vi "与副屏通信master.vi"() -> ()   [LabVIEW 2016, in "斯坦道多参数.lvlib"]
uses:
  <vilib>/NI/Modbus Library/API/Wrapper/Create TCP Master.vi
  <vilib>/NI/Modbus Library/API/master/Modbus Master.lvclass
  <vilib>/NI/Modbus Library/API/Wrapper/API Main.lvlib
  <vilib>/ptbypt/NI_PtbyPt.lvlib
panel:
  out "副屏启动命令":u16
  in  "停止 2":bool
  out "read values 2":u16[](array[numeric])
  in  "registers to write 2":u16[](array[numeric])
  out "error out 2":errorcluster caption="error out"
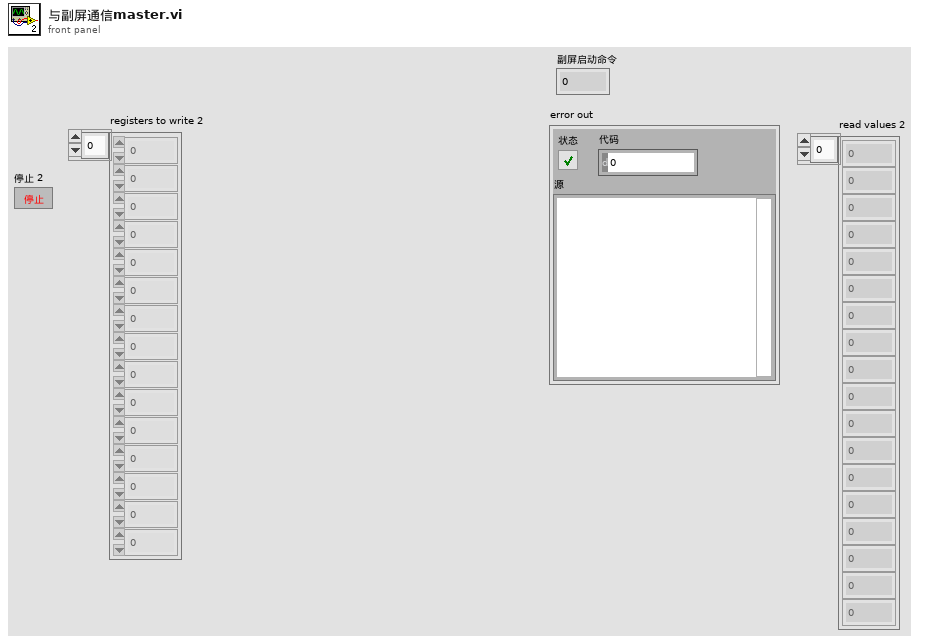
[diagram p1: front panel]
types:
  T1 = enum32{"Bad", "Idle", "Run top level", "Running"}
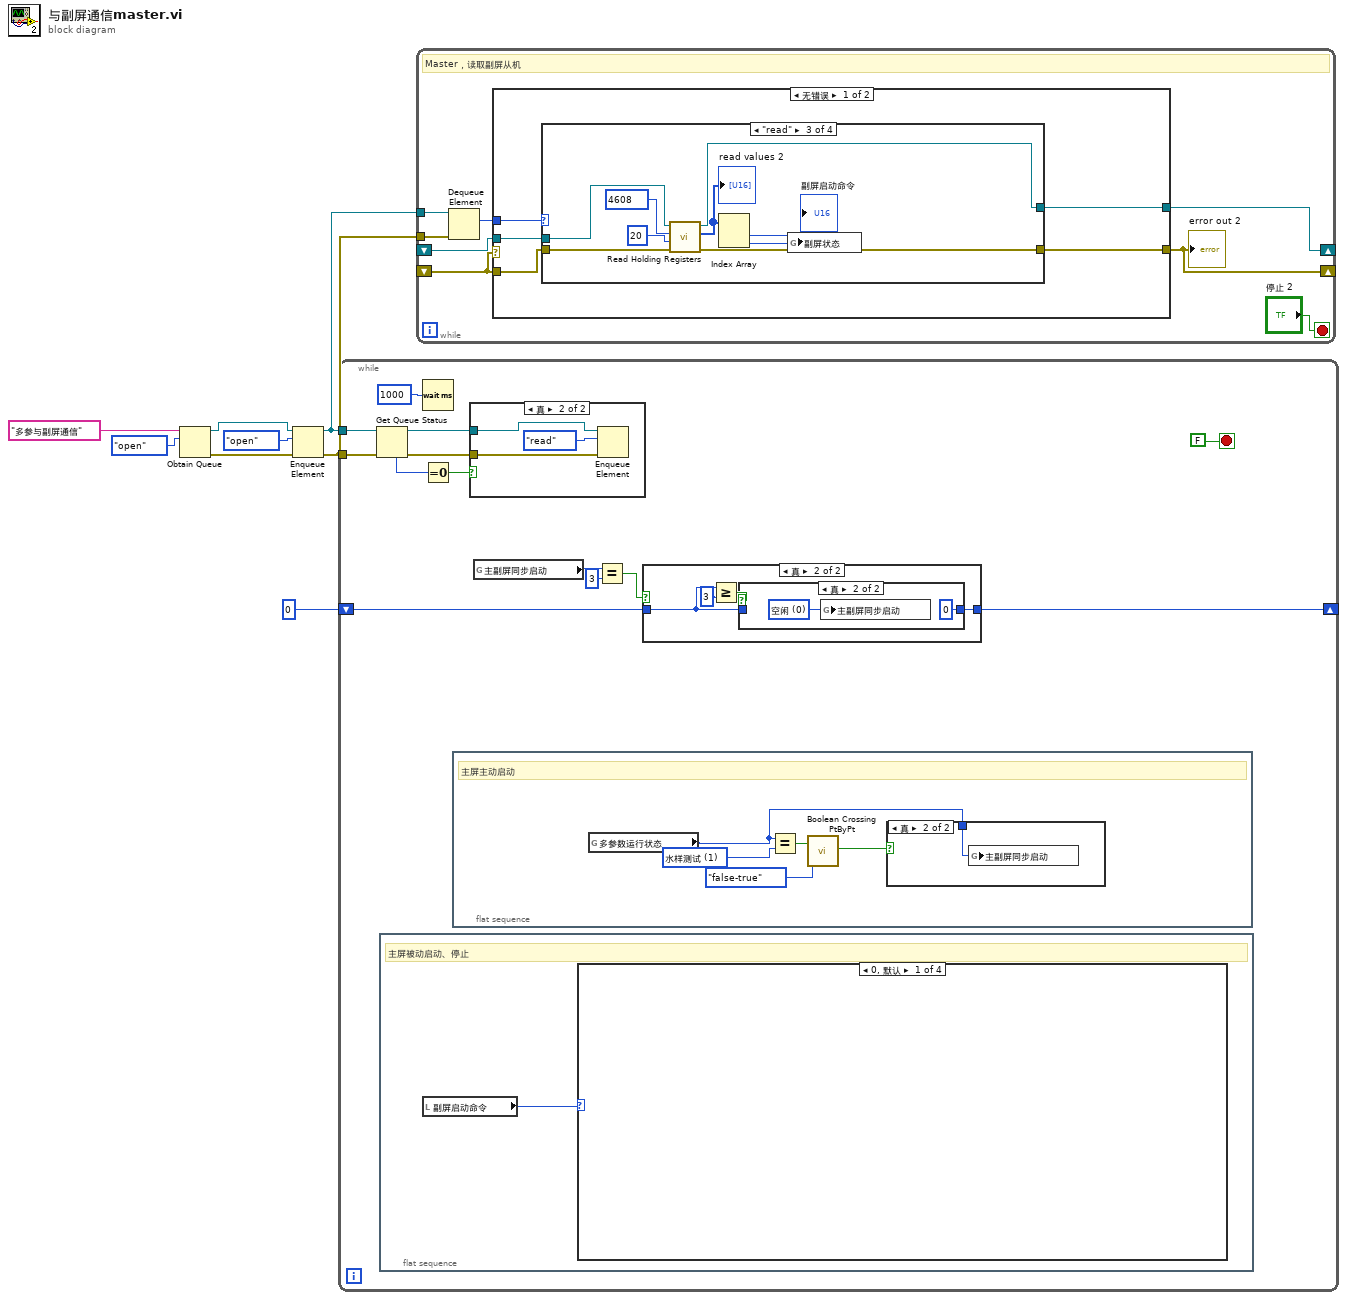
[diagram p0: block diagram]
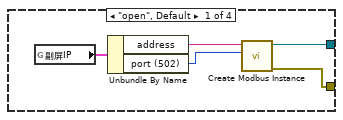
[diagram p2: hidden frame]
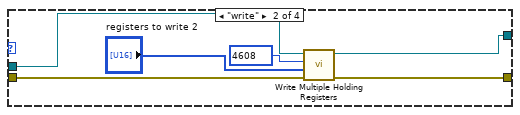
[diagram p3: hidden frame]
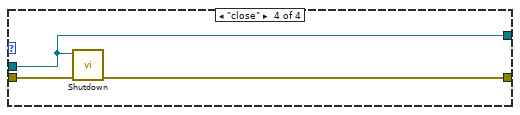
[diagram p4: hidden frame]
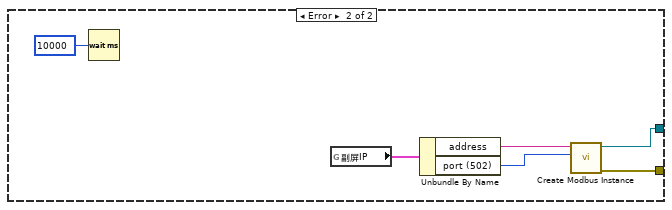
[diagram p5: hidden frame]
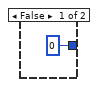
[diagram p6: hidden frame]
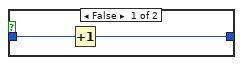
[diagram p7: hidden frame]
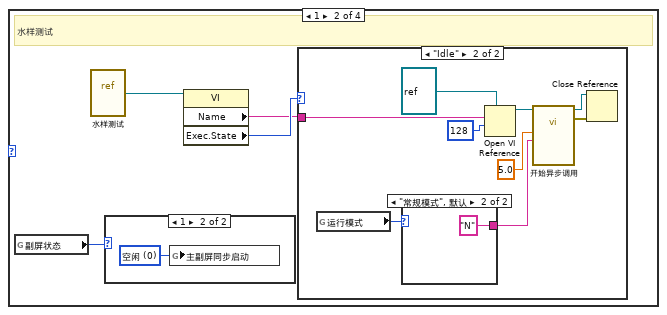
[diagram p8: hidden frame]
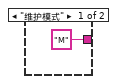
[diagram p11: hidden frame]
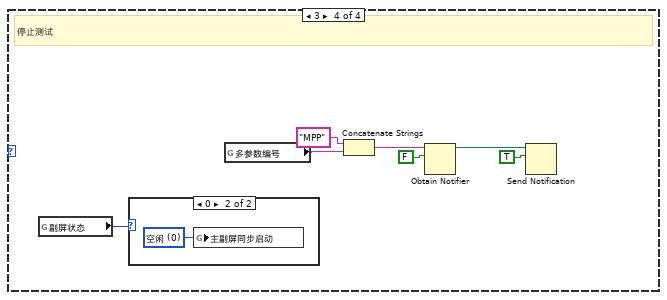
[diagram p13: hidden frame]
diagram:
  n1 = Obtain Queue(name (unnamed)="多参与副屏通信" ("名称（未命名）"), element data type=enum16{"open", "write", "read", "close"}."open") -> (queue out=w5:refnum<queue>, error out=w6:errorcluster)  [unwired: 3 in, 1 out]
  n2 = Enqueue Element(queue=w5, element=enum16{"open", "write", "read", "close"}."open", error in (no error)=w6) -> (queue out=w3:refnum<queue>, error out=w2:errorcluster)  [unwired: 1 in, 1 out]
  n3 = while {
    tunnel: w3 -> [w15]
    tunnel: w2 -> [w14]
    shift-right: [w9] -> _
    shift-left: u32 0 ("等待时间（毫秒）") -> [w10]
    stop <- FALSE stop-if-true
    n4 = Get Queue Status(queue=w15, error in (no error)=w14) -> (queue out=w17:refnum<queue>, error out=w18:errorcluster, # elements in queue=w16:i32)  [unwired: 1 in, 5 out]
    n5 = flat-sequence {
      frame #0 {
        # "主屏被动启动、停止"
        n6 = local read "副屏启动命令"() -> (w31:u16)
        n7 = case shown="0, 默认" w31 {
          frame 0, Default {
          }
          frame 1 {
            # "水样测试"
            n8 = global read "多参数全局变量.vi" "副屏状态"() -> (w32:u16)
            n9 = vi-ref "水样测试.vi"() -> (w35:refnum<vi>)
            n10 = case shown="1" w32 {
              frame 0, Default {
              }
              frame 1 {
                w36 = u16 0 items=["空闲", "水样测试", "标样核查", "停止"] ("主副屏同步启动")
                n11 = global write "多参数全局变量.vi" "主副屏同步启动"(w36) -> ()
              }
            }
            n12 = property class="VI"(reference=w35) -> ("Name"=w33:string, "Exec.State"=w34:T1)  [unwired: 1 in, 2 out]
            n13 = case shown="\"Idle\"" w34 {
              tunnel: w33 -> [_ w42]
              frame "Bad", Default {
              }
              frame "Idle" {
                n14 = global read "多参数全局变量.vi" "运行模式"() -> (w38:enum16{"维护模式", "常规模式", "应急模式", "质控模式"})
                n15 = case shown="\"常规模式\", 默认" w38 {
                  tunnel: ["M" ("数据标记表") "N" ("数据标记表")] -> w37
                  frame "维护模式" {
                  }
                  frame "常规模式", Default {
                  }
                }
                n16 = Open VI Reference(type specifier VI Refnum (for type only)=refnum<vi> refnum, vi path=w42, options=128 ("选项")) -> (vi reference=w43:refnum<vi>)  [unwired: 3 in, 1 out]
                n17 = call-by-ref "开始异步调用"(reference=w43, "数据标记表"=w37, "水样测试时间"=5.0) -> (reference out=w44:refnum<vi>, error out=w45:errorcluster)  [unwired: 11 in]
                n18 = Close Reference(reference=w44, error in (no error)=w45) -> ()  [unwired: 1 out]
              }
            }
          }
          frame 2 {
            # "标样核查"
          }
          frame 3 {
            # "停止测试"
            n19 = global read "多参数全局变量.vi" "副屏状态"() -> (w48:u16)
            n20 = case shown="0" w48 {
              frame 1, Default {
              }
              frame 0 {
                w55 = u16 0 items=["空闲", "水样测试", "标样核查", "停止"] ("主副屏同步启动")
                n21 = global write "多参数全局变量.vi" "主副屏同步启动"(w55) -> ()
              }
            }
            n22 = global read "多参数全局变量.vi" "多参数编号"() -> (w51:string)
            n23 = Concatenate Strings("MPP" ("名称（未命名）"), w51) -> (w52:string)
            n24 = Obtain Notifier(name (unnamed)=w52, notification data type=FALSE) -> (notifier out=w49:refnum<notifier>)  [unwired: 2 in, 2 out]
            n25 = Send Notification(notification=TRUE ("通知"), notifier=w49) -> ()  [unwired: 1 in, 2 out]
          }
        }
      }
    }
    n26 = Wait (ms)(milliseconds to wait=u32 1000 ("等待时间（毫秒）")) -> ()  [unwired: 1 out]
    n27 = Equal To 0?(x=w16) -> (x = 0?=w19:bool)
    n28 = flat-sequence {
      frame #0 {
        w58 = u16 1 items=["空闲", "水样测试", "标样核查"] ("多参数运行状态")
        # "主屏主动启动"
        n29 = global read "多参数全局变量.vi" "多参数运行状态"() -> (w56:u16)
        n30 = Equal?(x=w56, y=w58) -> (x = y?=w59:bool)
        n31 = call <vilib>:"Boolean Crossing PtByPt.vi"("direction"=enum16{"either", "false-true", "true-false"}."false-true", "input"=w59) -> ("crossing"=w57:bool)  [unwired: 1 in]
        n32 = case shown="真" w57 {
          tunnel: w56 -> [_ w61]
          frame False {
          }
          frame True {
            n33 = global write "多参数全局变量.vi" "主副屏同步启动"(w61) -> ()
          }
        }
      }
    }
    n34 = case shown="真" w19 {
      tunnel: w17 -> [_ w63]
      tunnel: w18 -> [_ w62]
      frame False {
      }
      frame True {
        n35 = Enqueue Element(queue=w63, element=enum16{"open", "write", "read", "close"}."read", error in (no error)=w62) -> ()  [unwired: 1 in, 3 out]
      }
    }
    n36 = global read "多参数全局变量.vi" "主副屏同步启动"() -> (w13:u16)
    n37 = Equal?(x=w13, y=u16 3) -> (x = y?=w11:bool)
    n38 = case shown="真" w11 {
      tunnel: w10 -> [_ w25]
      tunnel: [u32 0 w26] -> w9
      frame False {
      }
      frame True {
        n39 = Greater Or Equal?(x=w25, y=u32 3) -> (x >= y?=w23:bool)
        n40 = case shown="真" w23 {
          tunnel: [w28 u32 0] -> w26
          tunnel: w25 -> [w27 _]
          frame False {
            n41 = Increment(x=w27) -> (x+1=w28:u32)
          }
          frame True {
            w30 = u16 0 items=["空闲", "水样测试", "标样核查", "停止"] ("主副屏同步启动")
            n42 = global write "多参数全局变量.vi" "主副屏同步启动"(w30) -> ()
          }
        }
      }
    }
  }
  n43 = while {
    shift-right: [w69] -> _
    shift-left: _ -> [w71]
    shift-right: [w70] -> _
    shift-left: _ -> [w68]
    tunnel: w3 -> [w67]
    tunnel: w2 -> [w66]
    stop <- "停止 2" stop-if-true
    # "Master，读取副屏从机"
    n44 = Dequeue Element(queue=w67, error in (no error)=w66) -> (element=w65:enum16{"open", "write", "read", "close"})  [unwired: 1 in, 3 out]
    n45 = case shown="无错误" w68 {
      tunnel: w71 -> [w77 _]
      tunnel: w68 -> [w76 _]
      tunnel: [w75 w105] -> w70
      tunnel: [w74 w106] -> w69
      tunnel: w65 -> [w73 _]
      frame No Error {
        n46 = case shown="\"read\"" w73 {
          tunnel: w77 -> [_ w88 w97 w100]
          tunnel: w76 -> [_ w86 w94 w99]
          tunnel: [w81 w83 w93 w98] -> w75
          tunnel: [w82 w84 w92 w100] -> w74
          frame "open", Default {
            n47 = global read "多参数全局变量.vi" "副屏IP"() -> (w80:cluster{"address":string, "port (502)":u16})
            n48 = Unbundle By Name(w80) -> ("address"=w79:string, "port (502)"=w78:u16)
            n49 = call-poly <vilib>:"Create Modbus Instance.vi"("port (502)"=w78, "address"=w79) -> ("error out"=w81:errorcluster, "TCP master instance"=w82:refnum<class "Modbus Master.lvclass">)  [unwired: 8 in]
          }
          frame "write" {
            n50 = call-dynamic "Write Multiple Holding Registers.vi"("error in"=w86, "registers to write"="registers to write 2", "starting address"=u16 4608 ("write starting address"), "Modbus master in"=w88) -> ("error out"=w83:errorcluster, "Modbus master out"=w84:refnum<class "Modbus Master.lvclass">)  [unwired: 6 in]
          }
          frame "read" {
            n51 = call-dynamic "Read Holding Registers.vi"("error in"=w94, "number of inputs"=u16 20 ("read count"), "starting address"=u16 4608 ("write starting address"), "Modbus master in"=w97) -> ("error out"=w93:errorcluster, "register values"=w91:u16[], "Modbus master out"=w92:refnum<class "Modbus Master.lvclass">)  [unwired: 5 in]
            "read values 2" <- w91
            n52 = Index Array(array=w91) -> (element #1=→"副屏启动命令":u16, element #2=w90:u16)  [unwired: 2 in]
            n53 = global write "多参数全局变量.vi" "副屏状态"(w90) -> ()
          }
          frame "close" {
            n54 = call-dynamic "Shutdown.vi"("error in"=w99, "Modbus master in"=w100) -> ("error out"=w98:errorcluster)  [unwired: 9 in]
          }
        }
      }
      frame Error {
        n55 = Wait (ms)(milliseconds to wait=u32 10000 ("等待时间（毫秒）")) -> ()  [unwired: 1 out]
        n56 = global read "多参数全局变量.vi" "副屏IP"() -> (w103:cluster{"address":string, "port (502)":u16})
        n57 = Unbundle By Name(w103) -> ("address"=w102:string, "port (502)"=w101:u16)
        n58 = call-poly <vilib>:"Create Modbus Instance.vi"("port (502)"=w101, "address"=w102) -> ("error out"=w105:errorcluster, "TCP master instance"=w106:refnum<class "Modbus Master.lvclass">)  [unwired: 8 in]
      }
    }
    "error out 2" <- w70
  }
